vi "LakeShore218_Main.vi"() -> ()   [LabVIEW 2019]
panel:
  out "status":bool
  out "appended array":dbl[](array[numeric])
  out "r1":dbl format="%_6g"
  out "r2":dbl format="%_6g"
  out "r3":dbl format="%_6g"
  out "r8":dbl format="%_6g"
  out "r7":dbl format="%_6g"
  out "r6":dbl format="%_6g"
  out "r5":dbl format="%_6g"
  out "r4":dbl format="%_6g"
  out "Sensor data":cluster{cluster{"X":dbl, "Y":dbl}[]}[](graph)
  in  "stop":bool
  in  "VISA":refnum<visa-resource-name>
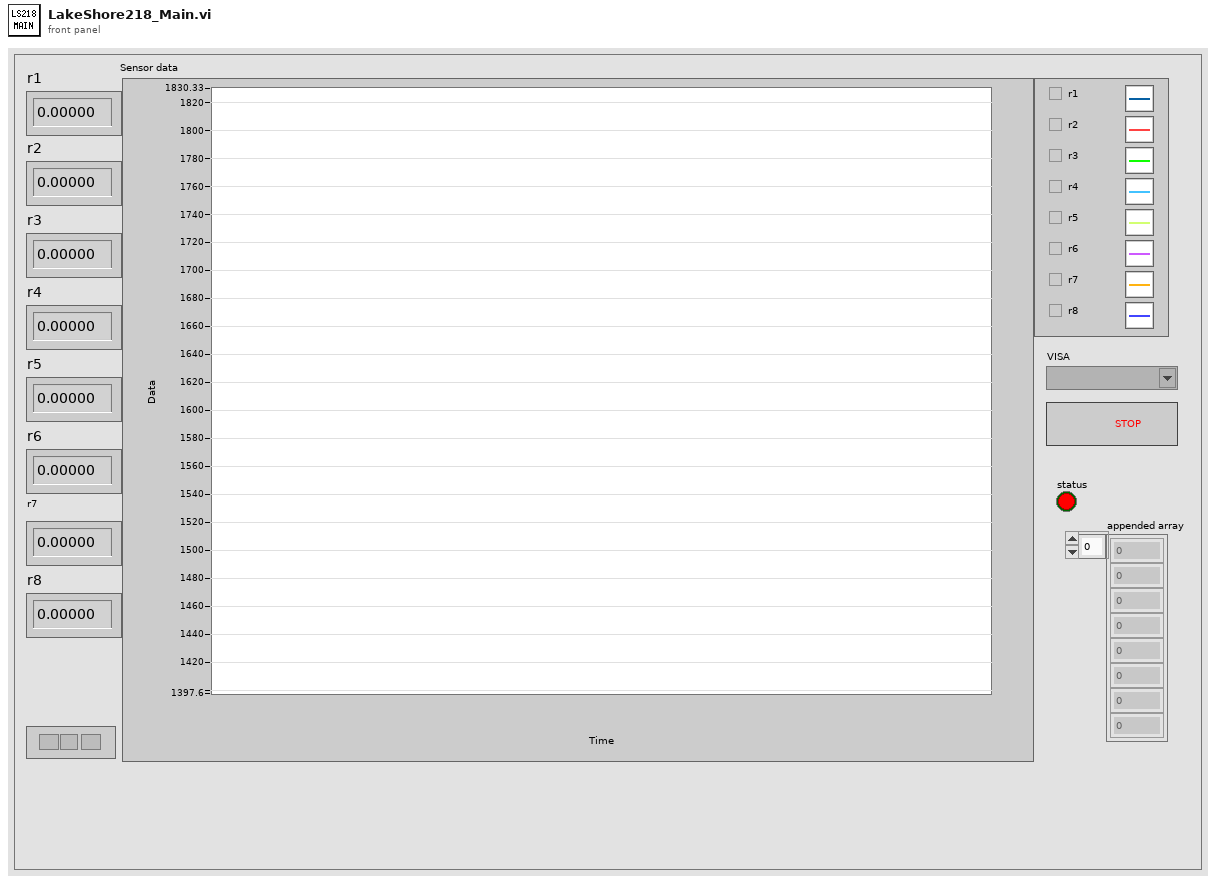
[diagram p1: front panel]
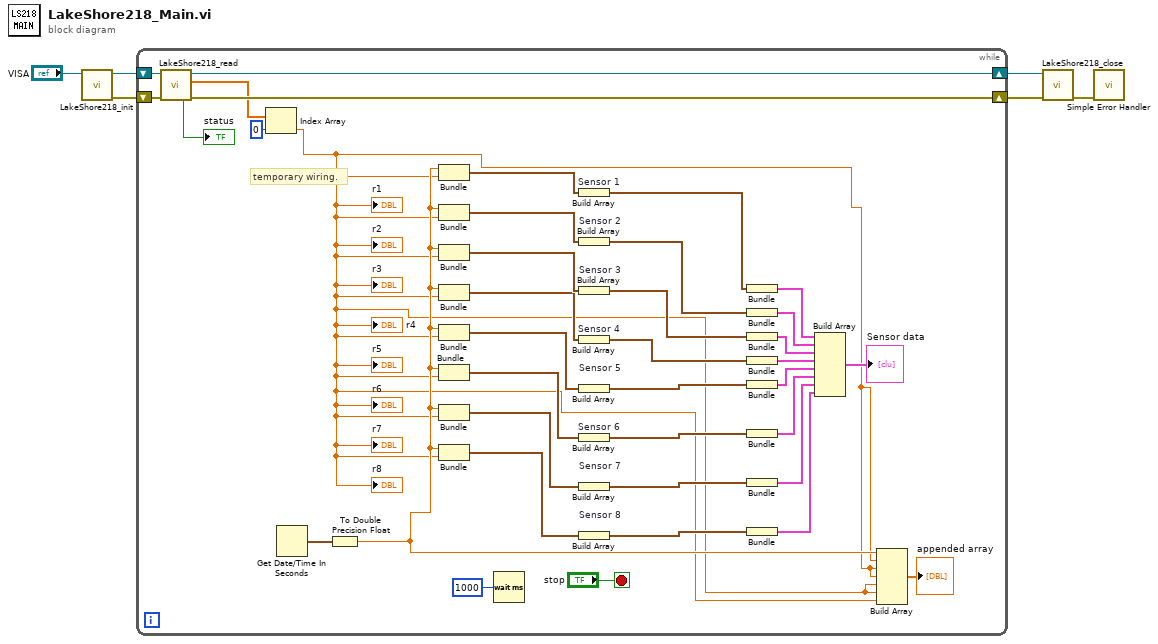
[diagram p0: block diagram]
diagram:
  n1 = call "LakeShore218_init.vi"("VISA in"="VISA") -> ("error out"=w6:errorcluster, "VISA out"=w5:refnum<visa-resource-name>)  [unwired: 9 in]
  n2 = while {
    shift-right: [w12] -> w3
    shift-left: w5 -> [w43]
    shift-right: [w11] -> w2
    shift-left: w6 -> [w44]
    stop <- "stop" stop-if-true
    # "temporary wiring."
    n3 = call "LakeShore218_read.vi"("error in"=w44, "VISA in"=w43) -> ("error out"=w11:errorcluster, "value_array"=w9:dbl[], "VISA out"=w12:refnum<visa-resource-name>, "status"=→"status":bool)  [unwired: 6 in]
    n4 = Index Array(array=w9, index=0) -> (element=w7:dbl)
    "r4" <- w7
    "r5" <- w7
    "r6" <- w7
    "r7" <- w7
    "r8" <- w7
    "r1" <- w7
    "r2" <- w7
    "r3" <- w7
    n5 = Get Date/Time In Seconds() -> (seconds since 1Jan1904=w32:timestamp)
    n6 = To Double Precision Float(number=w32) -> (double precision float=w14:dbl)
    n7 = Bundle(w14, w7) -> (w31:cluster{dbl, dbl})  [unwired: 1 in]
    n8 = Bundle(w14, w7) -> (w28:cluster{dbl, dbl})  [unwired: 1 in]
    n9 = Bundle(w14, w7) -> (w26:cluster{dbl, dbl})  [unwired: 1 in]
    n10 = Bundle(w14, w7) -> (w24:cluster{dbl, dbl})  [unwired: 1 in]
    n11 = Bundle(w14, w7) -> (w22:cluster{dbl, dbl})  [unwired: 1 in]
    n12 = Bundle(w14, w7) -> (w21:cluster{dbl, dbl})  [unwired: 1 in]
    n13 = Bundle(w14, w7) -> (w20:cluster{dbl, dbl})  [unwired: 1 in]
    n14 = Bundle(w14, w7) -> (w19:cluster{dbl, dbl})  [unwired: 1 in]
    n15 = Wait (ms)(milliseconds to wait=u32 1000) -> ()  [unwired: 1 out]
    n16 = Build Array "Sensor 1"(w31) -> (w40:cluster{dbl, dbl}[])
    n17 = Build Array "Sensor 2"(w28) -> (w39:cluster{dbl, dbl}[])
    n18 = Build Array "Sensor 3"(w26) -> (w38:cluster{dbl, dbl}[])
    n19 = Build Array "Sensor 4"(w24) -> (w37:cluster{dbl, dbl}[])
    n20 = Build Array "Sensor 5"(w22) -> (w36:cluster{dbl, dbl}[])
    n21 = Build Array "Sensor 6"(w21) -> (w35:cluster{dbl, dbl}[])
    n22 = Build Array "Sensor 7"(w20) -> (w34:cluster{dbl, dbl}[])
    n23 = Build Array "Sensor 8"(w19) -> (w33:cluster{dbl, dbl}[])
    n24 = Bundle(w40) -> (w30:cluster{cluster{dbl, dbl}[]})  [unwired: 1 in]
    n25 = Bundle(w39) -> (w27:cluster{cluster{dbl, dbl}[]})  [unwired: 1 in]
    n26 = Bundle(w38) -> (w25:cluster{cluster{dbl, dbl}[]})  [unwired: 1 in]
    n27 = Bundle(w37) -> (w23:cluster{cluster{dbl, dbl}[]})  [unwired: 1 in]
    n28 = Bundle(w36) -> (w18:cluster{cluster{dbl, dbl}[]})  [unwired: 1 in]
    n29 = Bundle(w35) -> (w17:cluster{cluster{dbl, dbl}[]})  [unwired: 1 in]
    n30 = Bundle(w34) -> (w16:cluster{cluster{dbl, dbl}[]})  [unwired: 1 in]
    n31 = Bundle(w33) -> (w15:cluster{cluster{dbl, dbl}[]})  [unwired: 1 in]
    n32 = Build Array(w30, w27, w25, w23, w18, w17, w16, w15) -> (→"Sensor data":cluster{cluster{dbl, dbl}[]}[])
    n33 = Build Array(w14, w7, w7, w7, w7, w7, w7) -> (→"appended array":dbl[])
  }
  n34 = call "LakeShore218_close.vi"("error in"=w2, "VISA in"=w3) -> ("error out"=w1:errorcluster)  [unwired: 9 in]
  n35 = call <vilib>:"Simple Error Handler.vi"("error in (no error)"=w1) -> ()  [unwired: 4 in, 5 out]
